vi "UTC Time to LabVIEW Time.vi"(5 "UTC Time (ns)":u64) -> (2 "LabVIEW Time (s)":timestamp)   [LabVIEW 2021, in "CIFUtilities.lvlib"]
uses:
  CIFUtilities.lvlib
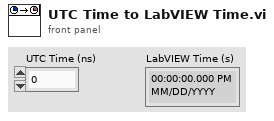
[diagram p1: front panel]
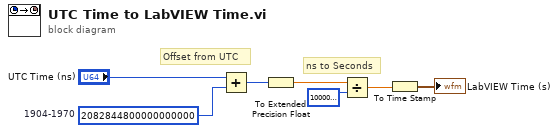
[diagram p0: block diagram]
diagram:
  w1 = u64 2082844800000000000  # 1904-1970
  # "Offset from UTC"
  # "ns to Seconds"
  n1 = Add(x="UTC Time (ns)", y=w1) -> (x+y=w2:u64)
  n2 = To Extended Precision Float(1:w2) -> (0:w3:ext)
  n3 = Divide(x=w3, y=u64 1000000000) -> (x/y=w7:ext)
  n4 = To Time Stamp(1:w7) -> (0:→"LabVIEW Time (s)":timestamp)
